vi "example_02_convert.vi"() -> ()   [LabVIEW 2015, in "lv-unit-conversion.lvlib"]
uses:
  lv-unit-conversion.lvlib
  public/_controls/unit.ctl
panel:
  out "error out":errorcluster
  in  "units []":T1[](array[typedef])=[{"symbol"="%", "name"="percent", "dimension"="1", "is_si_unit"=TRUE, "category"="atom-allowed", "base_unit"="Euc", "conversion_reference"="NIST-SI", "is_exact"=TRUE, "a"=0.0, "b"=0.01, "c"=1.0, "d"=0.0, "underlying_def"="1/100 Euc", "description"="Parts per hundred. \n\t\t\t\tThis is one of the few symbols which can be used with multiple unit classes. \n\t\t\t\tIt can be used with each class that represent a ratio of like quantities (e.g., mass per mass).\n\t\t\t"}, {"symbol"="ppk", "name"="part per thousand", "dimension"="1", "is_si_unit"=TRUE, "category"="atom", "base_unit"="Euc", "conversion_reference"="DEFINITION", "is_exact"=TRUE, "a"=0.0, "b"=0.001, "c"=1.0, "d"=0.0, "underlying_def"="", "description"="A ratio of values divided by 1000 where the original values were in the same units."}, {"symbol"="ppm", "name"="part per million", "dimension"="1", "is_si_unit"=TRUE, "category"="atom", "base_unit"="Euc", "conversion_reference"="DEFINITION", "is_exact"=TRUE, "a"=0.0, "b"=1e-06, "c"=1.0, "d"=0.0, "underlying_def"="", "description"="A ratio of values divided by 1E6 where the original values were in the same units."}, {"symbol"="Euc", "name"="euclid", "dimension"="1", "is_si_unit"=TRUE, "category"="atom-allowed", "base_unit"="", "conversion_reference"="", "is_exact"=FALSE, "a"=0.0, "b"=0.0, "c"=0.0, "d"=0.0, "underlying_def"="", "description"="A dimensionless unit of proportion, named after the Greek mathematician, Euclid. \n\t\t\t\tIt represents the SI implied unit of \"1\" which is sometimes called a \"dimensionless derived unit\".\n\t\t\t"}, {"symbol"="byte", "name"="byte", "dimension"="1", "is_si_unit"=TRUE, "category"="atom", "base_unit"="bit", "conversion_reference"="DEFINITION", "is_exact"=TRUE, "a"=0.0, "b"=8.0, "c"=1.0, "d"=0.0, "underlying_def"="8 bit", "description"="8 bit byte."}, {"symbol"="bit", "name"="bit", "dimension"="1", "is_si_unit"=TRUE, "category"="atom-allowed", "base_unit"="", "conversion_reference"="", "is_exact"=FALSE, "a"=0.0, "b"=0.0, "c"=0.0, "d"=0.0, "underlying_def"="Euc", "description"="A bit (a contraction of binary digit) is the basic unit of information in computing and \n\t\t\t\ttelecommunications. \n\t\t\t\tA bit can have only two values: either 1 or 0.\n\t\t\t"}, {"symbol"="%[mass]", "name"="percent [mass basis]", "dimension"="1", "is_si_unit"=TRUE, "category"="atom", "base_unit"="kg/kg", "conversion_reference"="DEFINITION", "is_exact"=TRUE, "a"=0.0, "b"=0.01, "c"=1.0, "d"=0.0, "underlying_def"="", "description"="The percent of mass relative to mass. \n\t\t\t\tThat is, mass divided by mass divided 100 where the original mass values were in the same units.\n\t\t\t"}, {"symbol"="ppm[mass]", "name"="part per million [mass basis]", "dimension"="1", "is_si_unit"=TRUE, "category"="atom", "base_unit"="kg/kg", "conversion_reference"="DEFINITION", "is_exact"=TRUE, "a"=0.0, "b"=1e-06, "c"=1.0, "d"=0.0, "underlying_def"="1E-6 kg/kg", "description"="The parts per million of mass relative to mass. \n\t\t\t\tThat is, mass divided by mass divided by 1E6 where the original mass values were in the same units.\n\t\t\t"}, {"symbol"="%[area]", "name"="percent [area basis]", "dimension"="1", "is_si_unit"=TRUE, "category"="atom", "base_unit"="m2/m2", "conversion_reference"="DERIVED", "is_exact"=TRUE, "a"=0.0, "b"=0.01, "c"=1.0, "d"=0.0, "underlying_def"="", "description"=""}, {"symbol"="%[vol]", "name"="percent [volume basis]", "dimension"="1", "is_si_unit"=TRUE, "category"="atom", "base_unit"="m3/m3", "conversion_reference"="DEFINITION", "is_exact"=TRUE, "a"=0.0, "b"=0.01, "c"=1.0, "d"=0.0, "underlying_def"="1/100 m3/m3", "description"="The percent of volume relative to volume That is, volume divided by volume divided by 100 where the \n\t\t\t\toriginal volume values were in the same units.\n\t\t\t"}, {"symbol"="ppm[vol]", "name"="part per million [volume basis]", "dimension"="1", "is_si_unit"=TRUE, "category"="atom", "base_unit"="m3/m3", "conversion_reference"="DEFINITION", "is_exact"=TRUE, "a"=0.0, "b"=1e-06, "c"=1.0, "d"=0.0, "underlying_def"="1E-6 m3/m3", "description"="The parts per million of volume relative to volume That is, volume divided by volume divided by 1E6 \n\t\t\t\twhere the original volume values were in the same units.\n\t\t\t"}, {"symbol"="%[molar]", "name"="percent [molar basis]", "dimension"="1", "is_si_unit"=TRUE, "category"="atom", "base_unit"="mol/mol", "conversion_reference"="DERIVED", "is_exact"=TRUE, "a"=0.0, "b"=0.01, "c"=1.0, "d"=0.0, "underlying_def"="", "description"=""}, {"symbol"="(bbl/d)/(bbl/d)", "name"="(barrel per day) per (barrel per day)", "dimension"="1", "is_si_unit"=TRUE, "category"="derived", "base_unit"="(m3/s)/(m3/s)", "conversion_reference"="DERIVED", "is_exact"=TRUE, "a"=0.0, "b"=1.0, "c"=1.0, "d"=0.0, "underlying_def"="", "description"=""}, {"symbol"="(m3/d)/(m3/d)", "name"="(cubic metre per day) per (cubic metre per day)", "dimension"="1", "is_si_unit"=TRUE, "category"="derived", "base_unit"="(m3/s)/(m3/s)", "conversion_reference"="DERIVED", "is_exact"=TRUE, "a"=0.0, "b"=1.0, "c"=1.0, "d"=0.0, "underlying_def"="", "description"=""}, {"symbol"="1E6 (ft3/d)/(bbl/d)", "name"="(million cubic foot per day) per (barrel per day)", "dimension"="1", "is_si_unit"=TRUE, "category"="derived", "base_unit"="(m3/s)/(m3/s)", "conversion_reference"="DERIVED", "is_exact"=TRUE, "a"=0.0, "b"=28316.846592, "c"=0.158987294928, "d"=0.0, "underlying_def"="", "description"=""}, {"symbol"="(m3/s)/(m3/s)", "name"="(cubic metre per second) per (cubic metre per second)", "dimension"="1", "is_si_unit"=TRUE, "category"="derived", "base_unit"="", "conversion_reference"="", "is_exact"=FALSE, "a"=0.0, "b"=0.0, "c"=0.0, "d"=0.0, "underlying_def"="Euc", "description"=""}, {"symbol"="kg/kg", "name"="kilogram per kilogram", "dimension"="1", "is_si_unit"=TRUE, "category"="derived", "base_unit"="", "conversion_reference"="", "is_exact"=FALSE, "a"=0.0, "b"=0.0, "c"=0.0, "d"=0.0, "underlying_def"="Euc", "description"=""}, {"symbol"="m/m", "name"="metre per metre", "dimension"="1", "is_si_unit"=TRUE, "category"="derived", "base_unit"="", "conversion_reference"="", "is_exact"=FALSE, "a"=0.0, "b"=0.0, "c"=0.0, "d"=0.0, "underlying_def"="Euc", "description"=""}, {"symbol"="m2/m2", "name"="square metre per square metre", "dimension"="1", "is_si_unit"=TRUE, "category"="derived", "base_unit"="", "conversion_reference"="", "is_exact"=FALSE, "a"=0.0, "b"=0.0, "c"=0.0, "d"=0.0, "underlying_def"="Euc", "description"=""}, {"symbol"="m3/m3", "name"="cubic metre per cubic metre", "dimension"="1", "is_si_unit"=TRUE, "category"="derived", "base_unit"="", "conversion_reference"="", "is_exact"=FALSE, "a"=0.0, "b"=0.0, "c"=0.0, "d"=0.0, "underlying_def"="Euc", "description"=""}, {"symbol"="mol/mol", "name"="mole per mole", "dimension"="1", "is_si_unit"=TRUE, "category"="derived", "base_unit"="", "conversion_reference"="", "is_exact"=FALSE, "a"=0.0, "b"=0.0, "c"=0.0, "d"=0.0, "underlying_def"="Euc", "description"=""}, {"symbol"="N/N", "name"="newton per newton", "dimension"="1", "is_si_unit"=TRUE, "category"="derived", "base_unit"="", "conversion_reference"="", "is_exact"=FALSE, "a"=0.0, "b"=0.0, "c"=0.0, "d"=0.0, "underlying_def"="Euc", "description"=""}, {"symbol"="s/s", "name"="second per second", "dimension"="1", "is_si_unit"=TRUE, "category"="derived", "base_unit"="", "conversion_reference"="", "is_exact"=FALSE, "a"=0.0, "b"=0.0, "c"=0.0, "d"=0.0, "underlying_def"="Euc", "description"=""}, {"symbol"="W/W", "name"="watt per watt", "dimension"="1", "is_si_unit"=TRUE, "category"="derived", "base_unit"="", "conversion_reference"="", "is_exact"=FALSE, "a"=0.0, "b"=0.0, "c"=0.0, "d"=0.0, "underlying_def"="Euc", "description"=""}, {"symbol"="g/kg", "name"="gram per kilogram", "dimension"="1", "is_si_unit"=TRUE, "category"="derived", "base_unit"="kg/kg", "conversion_reference"="DERIVED", "is_exact"=TRUE, "a"=0.0, "b"=0.001, "c"=1.0, "d"=0.0, "underlying_def"="", "description"=""}, {"symbol"="g/t", "name"="gram per tonne", "dimension"="1", "is_si_unit"=TRUE, "category"="derived", "base_unit"="kg/kg", "conversion_reference"="DERIVED", "is_exact"=TRUE, "a"=0.0, "b"=1e-06, "c"=1.0, "d"=0.0, "underlying_def"="", "description"=""}, {"symbol"="kg/sack[94lbm]", "name"="kilogram per 94-pound-sack", "dimension"="1", "is_si_unit"=TRUE, "category"="derived", "base_unit"="kg/kg", "conversion_reference"="DERIVED", "is_exact"=TRUE, "a"=0.0, "b"=1.0, "c"=42.63768278, "d"=0.0, "underlying_def"="", "description"=""}, {"symbol"="kg/t", "name"="kilogram per tonne", "dimension"="1", "is_si_unit"=TRUE, "category"="derived", "base_unit"="kg/kg", "conversion_reference"="DERIVED", "is_exact"=TRUE, "a"=0.0, "b"=0.001, "c"=1.0, "d"=0.0, "underlying_def"="", "description"=""}, {"symbol"="mg/g", "name"="milligram per gram", "dimension"="1", "is_si_unit"=TRUE, "category"="derived", "base_unit"="kg/kg", "conversion_reference"="DERIVED", "is_exact"=TRUE, "a"=0.0, "b"=0.001, "c"=1.0, "d"=0.0, "underlying_def"="", "description"=""}, {"symbol"="mg/kg", "name"="milligram per kilogram", "dimension"="1", "is_si_unit"=TRUE, "category"="derived", "base_unit"="kg/kg", "conversion_reference"="DERIVED", "is_exact"=TRUE, "a"=0.0, "b"=1e-06, "c"=1.0, "d"=0.0, "underlying_def"="", "description"=""}, {"symbol"="ng/g", "name"="nanogram per gram", "dimension"="1", "is_si_unit"=TRUE, "category"="derived", "base_unit"="kg/kg", "conversion_reference"="DERIVED", "is_exact"=TRUE, "a"=0.0, "b"=1e-09, "c"=1.0, "d"=0.0, "underlying_def"="", "description"=""}, {"symbol"="ng/mg", "name"="nanogram per milligram", "dimension"="1", "is_si_unit"=TRUE, "category"="derived", "base_unit"="kg/kg", "conversion_reference"="DERIVED", "is_exact"=TRUE, "a"=0.0, "b"=1e-06, "c"=1.0, "d"=0.0, "underlying_def"="", "description"=""}, {"symbol"="ug/g", "name"="microgram per gram", "dimension"="1", "is_si_unit"=TRUE, "category"="derived", "base_unit"="kg/kg", "conversion_reference"="DERIVED", "is_exact"=TRUE, "a"=0.0, "b"=1e-06, "c"=1.0, "d"=0.0, "underlying_def"="", "description"=""}, {"symbol"="ug/mg", "name"="microgram per milligram", "dimension"="1", "is_si_unit"=TRUE, "category"="derived", "base_unit"="kg/kg", "conversion_reference"="DERIVED", "is_exact"=TRUE, "a"=0.0, "b"=0.001, "c"=1.0, "d"=0.0, "underlying_def"="", "description"=""}, {"symbol"="0.01 ft/ft", "name"="foot per hundred foot", "dimension"="1", "is_si_unit"=TRUE, "category"="derived", "base_unit"="m/m", "conversion_reference"="DERIVED", "is_exact"=TRUE, "a"=0.0, "b"=0.01, "c"=1.0, "d"=0.0, "underlying_def"="", "description"=""}, {"symbol"="1/30 m/m", "name"="metre per thirty metre", "dimension"="1", "is_si_unit"=TRUE, "category"="derived", "base_unit"="m/m", "conversion_reference"="DERIVED", "is_exact"=TRUE, "a"=0.0, "b"=1.0, "c"=30.0, "d"=0.0, "underlying_def"="", "description"=""}, {"symbol"="ft/ft", "name"="foot per foot", "dimension"="1", "is_si_unit"=TRUE, "category"="derived", "base_unit"="m/m", "conversion_reference"="DERIVED", "is_exact"=TRUE, "a"=0.0, "b"=1.0, "c"=1.0, "d"=0.0, "underlying_def"="", "description"=""}, {"symbol"="ft/in", "name"="foot per inch", "dimension"="1", "is_si_unit"=TRUE, "category"="derived", "base_unit"="m/m", "conversion_reference"="DERIVED", "is_exact"=TRUE, "a"=0.0, "b"=12.0, "c"=1.0, "d"=0.0, "underlying_def"="", "description"=""}, {"symbol"="ft/m", "name"="foot per metre", "dimension"="1", "is_si_unit"=TRUE, "category"="derived", "base_unit"="m/m", "conversion_reference"="DERIVED", "is_exact"=TRUE, "a"=0.0, "b"=0.3048, "c"=1.0, "d"=0.0, "underlying_def"="", "description"=""}, {"symbol"="ft/mi", "name"="foot per mile", "dimension"="1", "is_si_unit"=TRUE, "category"="derived", "base_unit"="m/m", "conversion_reference"="DERIVED", "is_exact"=TRUE, "a"=0.0, "b"=1.0, "c"=5280.0, "d"=0.0, "underlying_def"="", "description"=""}, {"symbol"="km/cm", "name"="kilometre per centimetre", "dimension"="1", "is_si_unit"=TRUE, "category"="derived", "base_unit"="m/m", "conversion_reference"="DERIVED", "is_exact"=TRUE, "a"=0.0, "b"=100000.0, "c"=1.0, "d"=0.0, "underlying_def"="", "description"=""}, {"symbol"="m/cm", "name"="metre per centimetre", "dimension"="1", "is_si_unit"=TRUE, "category"="derived", "base_unit"="m/m", "conversion_reference"="DERIVED", "is_exact"=TRUE, "a"=0.0, "b"=100.0, "c"=1.0, "d"=0.0, "underlying_def"="", "description"=""}, {"symbol"="m/km", "name"="metre per kilometre", "dimension"="1", "is_si_unit"=TRUE, "category"="derived", "base_unit"="m/m", "conversion_reference"="DERIVED", "is_exact"=TRUE, "a"=0.0, "b"=0.001, "c"=1.0, "d"=0.0, "underlying_def"="", "description"="Parts per thousand."}, {"symbol"="mi/in", "name"="mile per inch", "dimension"="1", "is_si_unit"=TRUE, "category"="derived", "base_unit"="m/m", "conversion_reference"="DERIVED", "is_exact"=TRUE, "a"=0.0, "b"=63360.0, "c"=1.0, "d"=0.0, "underlying_def"="", "description"=""}, {"symbol"="in2/ft2", "name"="square inch per square foot", "dimension"="1", "is_si_unit"=TRUE, "category"="derived", "base_unit"="m2/m2", "conversion_reference"="DERIVED", "is_exact"=TRUE, "a"=0.0, "b"=1.0, "c"=144.0, "d"=0.0, "underlying_def"="", "description"=""}, {"symbol"="in2/in2", "name"="square inch per square inch", "dimension"="1", "is_si_unit"=TRUE, "category"="derived", "base_unit"="m2/m2", "conversion_reference"="DERIVED", "is_exact"=TRUE, "a"=0.0, "b"=1.0, "c"=1.0, "d"=0.0, "underlying_def"="", "description"=""}, {"symbol"="mm2/mm2", "name"="square millimetre per square millimetre", "dimension"="1", "is_si_unit"=TRUE, "category"="derived", "base_unit"="m2/m2", "conversion_reference"="DERIVED", "is_exact"=TRUE, "a"=0.0, "b"=1.0, "c"=1.0, "d"=0.0, "underlying_def"="", "description"=""}, {"symbol"="0.001 bbl/ft3", "name"="barrel per thousand cubic foot", "dimension"="1", "is_si_unit"=TRUE, "category"="derived", "base_unit"="m3/m3", "conversion_reference"="DERIVED", "is_exact"=TRUE, "a"=0.0, "b"=0.000158987294928, "c"=0.028316846592, "d"=0.0, "underlying_def"="", "description"=""}, {"symbol"="0.001 bbl/m3", "name"="barrel per thousand cubic metre", "dimension"="1", "is_si_unit"=TRUE, "category"="derived", "base_unit"="m3/m3", "conversion_reference"="DERIVED", "is_exact"=TRUE, "a"=0.0, "b"=0.000158987294928, "c"=1.0, "d"=0.0, "underlying_def"="", "description"=""}, {"symbol"="0.001 gal[UK]/bbl", "name"="UK gallon per thousand barrel", "dimension"="1", "is_si_unit"=TRUE, "category"="derived", "base_unit"="m3/m3", "conversion_reference"="DERIVED", "is_exact"=TRUE, "a"=0.0, "b"=4.54609e-06, "c"=0.158987294928, "d"=0.0, "underlying_def"="", "description"=""}, {"symbol"="0.001 gal[UK]/gal[UK]", "name"="UK gallon per thousand UK gallon", "dimension"="1", "is_si_unit"=TRUE, "category"="derived", "base_unit"="m3/m3", "conversion_reference"="DERIVED", "is_exact"=TRUE, "a"=0.0, "b"=0.001, "c"=1.0, "d"=0.0, "underlying_def"="", "description"=""}, {"symbol"="0.001 gal[US]/bbl", "name"="US gallon per thousand barrel", "dimension"="1", "is_si_unit"=TRUE, "category"="derived", "base_unit"="m3/m3", "conversion_reference"="DERIVED", "is_exact"=TRUE, "a"=0.0, "b"=3.785411784e-06, "c"=0.158987294928, "d"=0.0, "underlying_def"="", "description"=""}, {"symbol"="0.001 gal[US]/ft3", "name"="US gallon per thousand cubic foot", "dimension"="1", "is_si_unit"=TRUE, "category"="derived", "base_unit"="m3/m3", "conversion_reference"="DERIVED", "is_exact"=TRUE, "a"=0.0, "b"=3.785411784e-06, "c"=0.028316846592, "d"=0.0, "underlying_def"="", "description"=""}, {"symbol"="0.001 gal[US]/gal[US]", "name"="US gallon per thousand US gallon", "dimension"="1", "is_si_unit"=TRUE, "category"="derived", "base_unit"="m3/m3", "conversion_reference"="DERIVED", "is_exact"=TRUE, "a"=0.0, "b"=0.001, "c"=1.0, "d"=0.0, "underlying_def"="", "description"=""}, {"symbol"="0.001 pt[UK]/bbl", "name"="UK pint per thousand barrel", "dimension"="1", "is_si_unit"=TRUE, "category"="derived", "base_unit"="m3/m3", "conversion_reference"="DERIVED", "is_exact"=TRUE, "a"=0.0, "b"=0.00056826125, "c"=158.987294928, "d"=0.0, "underlying_def"="", "description"=""}, {"symbol"="0.01 bbl/bbl", "name"="barrel per hundred barrel", "dimension"="1", "is_si_unit"=TRUE, "category"="derived", "base_unit"="m3/m3", "conversion_reference"="DERIVED", "is_exact"=TRUE, "a"=0.0, "b"=0.01, "c"=1.0, "d"=0.0, "underlying_def"="", "description"=""}, {"symbol"="0.1 gal[US]/bbl", "name"="US gallon per ten barrel", "dimension"="1", "is_si_unit"=TRUE, "category"="derived", "base_unit"="m3/m3", "conversion_reference"="DERIVED", "is_exact"=TRUE, "a"=0.0, "b"=0.0003785411784, "c"=0.158987294928, "d"=0.0, "underlying_def"="", "description"=""}, {"symbol"="0.1 L/bbl", "name"="litre per ten barrel", "dimension"="1", "is_si_unit"=TRUE, "category"="derived", "base_unit"="m3/m3", "conversion_reference"="DERIVED", "is_exact"=TRUE, "a"=0.0, "b"=0.001, "c"=1.58987294928, "d"=0.0, "underlying_def"="", "description"=""}, {"symbol"="0.1 pt[US]/bbl", "name"="US pint per ten barrel", "dimension"="1", "is_si_unit"=TRUE, "category"="derived", "base_unit"="m3/m3", "conversion_reference"="DERIVED", "is_exact"=TRUE, "a"=0.0, "b"=0.000473176473, "c"=1.58987294928, "d"=0.0, "underlying_def"="", "description"=""}, {"symbol"="1000 ft3/bbl", "name"="thousand cubic foot per barrel", "dimension"="1", "is_si_unit"=TRUE, "category"="derived", "base_unit"="m3/m3", "conversion_reference"="DERIVED", "is_exact"=TRUE, "a"=0.0, "b"=28.316846592, "c"=0.158987294928, "d"=0.0, "underlying_def"="", "description"=""}, {"symbol"="1000 m3/m3", "name"="thousand cubic metre per cubic metre", "dimension"="1", "is_si_unit"=TRUE, "category"="derived", "base_unit"="m3/m3", "conversion_reference"="DERIVED", "is_exact"=TRUE, "a"=0.0, "b"=1000.0, "c"=1.0, "d"=0.0, "underlying_def"="", "description"=""}, {"symbol"="1E-6 acre.ft/bbl", "name"="acre foot per million barrel", "dimension"="1", "is_si_unit"=TRUE, "category"="derived", "base_unit"="m3/m3", "conversion_reference"="DERIVED", "is_exact"=TRUE, "a"=0.0, "b"=19119.00672, "c"=2464298.1427778574, "d"=0.0, "underlying_def"="", "description"=""}, {"symbol"="1E6 bbl/(acre.ft)", "name"="million barrel per acre foot", "dimension"="1", "is_si_unit"=TRUE, "category"="derived", "base_unit"="m3/m3", "conversion_reference"="DERIVED", "is_exact"=TRUE, "a"=0.0, "b"=2464298142777.8574, "c"=19119006720.0, "d"=0.0, "underlying_def"="", "description"=""}, {"symbol"="1E-6 bbl/ft3", "name"="barrel per million cubic foot", "dimension"="1", "is_si_unit"=TRUE, "category"="derived", "base_unit"="m3/m3", "conversion_reference"="DERIVED", "is_exact"=TRUE, "a"=0.0, "b"=0.158987294928, "c"=28316.846592, "d"=0.0, "underlying_def"="", "description"=""}, {"symbol"="1E-6 bbl/m3", "name"="barrel per million cubic metre", "dimension"="1", "is_si_unit"=TRUE, "category"="derived", "base_unit"="m3/m3", "conversion_reference"="DERIVED", "is_exact"=TRUE, "a"=0.0, "b"=1.58987294928e-07, "c"=1.0, "d"=0.0, "underlying_def"="", "description"="barrel per million cubic metre"}, {"symbol"="1E6 ft3/(acre.ft)", "name"="million cubic foot per acre foot", "dimension"="1", "is_si_unit"=TRUE, "category"="derived", "base_unit"="m3/m3", "conversion_reference"="DERIVED", "is_exact"=TRUE, "a"=0.0, "b"=1439994240005.76, "c"=62726400000.0, "d"=0.0, "underlying_def"="", "description"=""}, {"symbol"="1E6 ft3/bbl", "name"="million cubic foot per barrel", "dimension"="1", "is_si_unit"=TRUE, "category"="derived", "base_unit"="m3/m3", "conversion_reference"="DERIVED", "is_exact"=TRUE, "a"=0.0, "b"=28316.846592, "c"=0.158987294928, "d"=0.0, "underlying_def"="", "description"=""}, {"symbol"="bbl/(acre.ft)", "name"="barrel per acre foot", "dimension"="1", "is_si_unit"=TRUE, "category"="derived", "base_unit"="m3/m3", "conversion_reference"="DERIVED", "is_exact"=TRUE, "a"=0.0, "b"=2464298.1427778574, "c"=19119006720.0, "d"=0.0, "underlying_def"="", "description"=""}, {"symbol"="bbl/bbl", "name"="barrel per barrel", "dimension"="1", "is_si_unit"=TRUE, "category"="derived", "base_unit"="m3/m3", "conversion_reference"="DERIVED", "is_exact"=TRUE, "a"=0.0, "b"=1.0, "c"=1.0, "d"=0.0, "underlying_def"="", "description"=""}, {"symbol"="bbl/ft3", "name"="barrel per cubic foot", "dimension"="1", "is_si_unit"=TRUE, "category"="derived", "base_unit"="m3/m3", "conversion_reference"="DERIVED", "is_exact"=TRUE, "a"=0.0, "b"=0.158987294928, "c"=0.028316846592, "d"=0.0, "underlying_def"="", "description"=""}, {"symbol"="bbl/m3", "name"="barrel per cubic metre", "dimension"="1", "is_si_unit"=TRUE, "category"="derived", "base_unit"="m3/m3", "conversion_reference"="DERIVED", "is_exact"=TRUE, "a"=0.0, "b"=0.158987294928, "c"=1.0, "d"=0.0, "underlying_def"="", "description"=""}, {"symbol"="cm3/cm3", "name"="cubic centimetre per cubic centimetre", "dimension"="1", "is_si_unit"=TRUE, "category"="derived", "base_unit"="m3/m3", "conversion_reference"="DERIVED", "is_exact"=TRUE, "a"=0.0, "b"=1.0, "c"=1.0, "d"=0.0, "underlying_def"="", "description"=""}, {"symbol"="cm3/L", "name"="cubic centimetre per litre", "dimension"="1", "is_si_unit"=TRUE, "category"="derived", "base_unit"="m3/m3", "conversion_reference"="DERIVED", "is_exact"=TRUE, "a"=0.0, "b"=0.001, "c"=1.0, "d"=0.0, "underlying_def"="", "description"=""}, {"symbol"="cm3/m3", "name"="cubic centimetre per cubic metre", "dimension"="1", "is_si_unit"=TRUE, "category"="derived", "base_unit"="m3/m3", "conversion_reference"="DERIVED", "is_exact"=TRUE, "a"=0.0, "b"=1e-06, "c"=1.0, "d"=0.0, "underlying_def"="", "description"="Part per million [mass per mass]"}, {"symbol"="dm3/m3", "name"="cubic decimetre per cubic metre", "dimension"="1", "is_si_unit"=TRUE, "category"="derived", "base_unit"="m3/m3", "conversion_reference"="DERIVED", "is_exact"=TRUE, "a"=0.0, "b"=0.001, "c"=1.0, "d"=0.0, "underlying_def"="", "description"=""}, {"symbol"="ft3/bbl", "name"="cubic foot per barrel", "dimension"="1", "is_si_unit"=TRUE, "category"="derived", "base_unit"="m3/m3", "conversion_reference"="DERIVED", "is_exact"=TRUE, "a"=0.0, "b"=0.028316846592, "c"=0.158987294928, "d"=0.0, "underlying_def"="", "description"=""}, {"symbol"="ft3/ft3", "name"="cubic foot per cubic foot", "dimension"="1", "is_si_unit"=TRUE, "category"="derived", "base_unit"="m3/m3", "conversion_reference"="DERIVED", "is_exact"=TRUE, "a"=0.0, "b"=1.0, "c"=1.0, "d"=0.0, "underlying_def"="", "description"=""}, {"symbol"="gal[UK]/ft3", "name"="UK gallon per cubic foot", "dimension"="1", "is_si_unit"=TRUE, "category"="derived", "base_unit"="m3/m3", "conversion_reference"="DERIVED", "is_exact"=TRUE, "a"=0.0, "b"=0.00454609, "c"=0.028316846592, "d"=0.0, "underlying_def"="", "description"=""}, {"symbol"="gal[US]/bbl", "name"="US gallon per barrel", "dimension"="1", "is_si_unit"=TRUE, "category"="derived", "base_unit"="m3/m3", "conversion_reference"="DERIVED", "is_exact"=TRUE, "a"=0.0, "b"=0.003785411784, "c"=0.158987294928, "d"=0.0, "underlying_def"="", "description"=""}, {"symbol"="gal[US]/ft3", "name"="US gallon per cubic foot", "dimension"="1", "is_si_unit"=TRUE, "category"="derived", "base_unit"="m3/m3", "conversion_reference"="DERIVED", "is_exact"=TRUE, "a"=0.0, "b"=0.003785411784, "c"=0.028316846592, "d"=0.0, "underlying_def"="", "description"=""}, {"symbol"="L/m3", "name"="litre per cubic metre", "dimension"="1", "is_si_unit"=TRUE, "category"="derived", "base_unit"="m3/m3", "conversion_reference"="DERIVED", "is_exact"=TRUE, "a"=0.0, "b"=0.001, "c"=1.0, "d"=0.0, "underlying_def"="", "description"=""}, {"symbol"="m3/(ha.m)", "name"="cubic metre per hectare metre", "dimension"="1", "is_si_unit"=TRUE, "category"="derived", "base_unit"="m3/m3", "conversion_reference"="DERIVED", "is_exact"=TRUE, "a"=0.0, "b"=0.0001, "c"=1.0, "d"=0.0, "underlying_def"="", "description"=""}, {"symbol"="m3/bbl", "name"="cubic metre per barrel", "dimension"="1", "is_si_unit"=TRUE, "category"="derived", "base_unit"="m3/m3", "conversion_reference"="DERIVED", "is_exact"=TRUE, "a"=0.0, "b"=1.0, "c"=0.158987294928, "d"=0.0, "underlying_def"="", "description"=""}, {"symbol"="mL/gal[UK]", "name"="millilitre per UK gallon", "dimension"="1", "is_si_unit"=TRUE, "category"="derived", "base_unit"="m3/m3", "conversion_reference"="DERIVED", "is_exact"=TRUE, "a"=0.0, "b"=1e-06, "c"=0.00454609, "d"=0.0, "underlying_def"="", "description"=""}, {"symbol"="mL/gal[US]", "name"="millilitre per US gallon", "dimension"="1", "is_si_unit"=TRUE, "category"="derived", "base_unit"="m3/m3", "conversion_reference"="DERIVED", "is_exact"=TRUE, "a"=0.0, "b"=1e-06, "c"=0.003785411784, "d"=0.0, "underlying_def"="", "description"=""}, {"symbol"="mL/mL", "name"="millilitre per millilitre", "dimension"="1", "is_si_unit"=TRUE, "category"="derived", "base_unit"="m3/m3", "conversion_reference"="DERIVED", "is_exact"=TRUE, "a"=0.0, "b"=1.0, "c"=1.0, "d"=0.0, "underlying_def"="", "description"=""}, {"symbol"="kgf/kgf", "name"="thousand gram-force per kilogram-force", "dimension"="1", "is_si_unit"=TRUE, "category"="derived", "base_unit"="N/N", "conversion_reference"="DERIVED", "is_exact"=TRUE, "a"=0.0, "b"=1.0, "c"=1.0, "d"=0.0, "underlying_def"="", "description"=""}, {"symbol"="lbf/lbf", "name"="pound-force per pound-force", "dimension"="1", "is_si_unit"=TRUE, "category"="derived", "base_unit"="N/N", "conversion_reference"="DERIVED", "is_exact"=TRUE, "a"=0.0, "b"=1.0, "c"=1.0, "d"=0.0, "underlying_def"="", "description"=""}, {"symbol"="ms/s", "name"="millisecond per second", "dimension"="1", "is_si_unit"=TRUE, "category"="derived", "base_unit"="s/s", "conversion_reference"="DERIVED", "is_exact"=TRUE, "a"=0.0, "b"=0.001, "c"=1.0, "d"=0.0, "underlying_def"="", "description"=""}, {"symbol"="Btu[IT]/(hp.h)", "name"="BTU per horsepower hour", "dimension"="1", "is_si_unit"=TRUE, "category"="derived", "base_unit"="W/W", "conversion_reference"="DERIVED", "is_exact"=TRUE, "a"=0.0, "b"=1055.05585262, "c"=2684519.537696173, "d"=0.0, "underlying_def"="", "description"=""}, {"symbol"="W/kW", "name"="watt per kilowatt", "dimension"="1", "is_si_unit"=TRUE, "category"="derived", "base_unit"="W/W", "conversion_reference"="DERIVED", "is_exact"=TRUE, "a"=0.0, "b"=0.001, "c"=1.0, "d"=0.0, "underlying_def"="", "description"=""}, {"symbol"="cEuc", "name"="centieuclid", "dimension"="1", "is_si_unit"=TRUE, "category"="prefixed", "base_unit"="Euc", "conversion_reference"="DERIVED", "is_exact"=TRUE, "a"=0.0, "b"=0.01, "c"=1.0, "d"=0.0, "underlying_def"="", "description"="Parts per hundred."}, {"symbol"="dEuc", "name"="decieuclid", "dimension"="1", "is_si_unit"=TRUE, "category"="prefixed", "base_unit"="Euc", "conversion_reference"="DERIVED", "is_exact"=TRUE, "a"=0.0, "b"=0.1, "c"=1.0, "d"=0.0, "underlying_def"="", "description"="Parts per ten."}, {"symbol"="EEuc", "name"="exaeuclid", "dimension"="1", "is_si_unit"=TRUE, "category"="prefixed", "base_unit"="Euc", "conversion_reference"="DERIVED", "is_exact"=TRUE, "a"=0.0, "b"=1e+18, "c"=1.0, "d"=0.0, "underlying_def"="", "description"="Million million million per part."}, {"symbol"="fEuc", "name"="femtoeuclid", "dimension"="1", "is_si_unit"=TRUE, "category"="prefixed", "base_unit"="Euc", "conversion_reference"="DERIVED", "is_exact"=TRUE, "a"=0.0, "b"=1e-15, "c"=1.0, "d"=0.0, "underlying_def"="", "description"="Parts per thousand million million."}, {"symbol"="GEuc", "name"="gigaeuclid", "dimension"="1", "is_si_unit"=TRUE, "category"="prefixed", "base_unit"="Euc", "conversion_reference"="DERIVED", "is_exact"=TRUE, "a"=0.0, "b"=1000000000.0, "c"=1.0, "d"=0.0, "underlying_def"="", "description"="Thousand million per part."}, {"symbol"="kEuc", "name"="kiloeuclid", "dimension"="1", "is_si_unit"=TRUE, "category"="prefixed", "base_unit"="Euc", "conversion_reference"="DERIVED", "is_exact"=TRUE, "a"=0.0, "b"=1000.0, "c"=1.0, "d"=0.0, "underlying_def"="", "description"="Thousand per part."}, {"symbol"="mEuc", "name"="millieuclid", "dimension"="1", "is_si_unit"=TRUE, "category"="prefixed", "base_unit"="Euc", "conversion_reference"="DERIVED", "is_exact"=TRUE, "a"=0.0, "b"=0.001, "c"=1.0, "d"=0.0, "underlying_def"="", "description"="Parts per thousand."}, {"symbol"="MEuc", "name"="megaeuclid", "dimension"="1", "is_si_unit"=TRUE, "category"="prefixed", "base_unit"="Euc", "conversion_reference"="DERIVED", "is_exact"=TRUE, "a"=0.0, "b"=1000000.0, "c"=1.0, "d"=0.0, "underlying_def"="", "description"="Million per part."}, {"symbol"="nEuc", "name"="nanoeuclid", "dimension"="1", "is_si_unit"=TRUE, "category"="prefixed", "base_unit"="Euc", "conversion_reference"="DERIVED", "is_exact"=TRUE, "a"=0.0, "b"=1e-09, "c"=1.0, "d"=0.0, "underlying_def"="", "description"="Parts per thousand million."}, {"symbol"="pEuc", "name"="picoeuclid", "dimension"="1", "is_si_unit"=TRUE, "category"="prefixed", "base_unit"="Euc", "conversion_reference"="DERIVED", "is_exact"=TRUE, "a"=0.0, "b"=1e-12, "c"=1.0, "d"=0.0, "underlying_def"="", "description"="Parts per million million."}, {"symbol"="TEuc", "name"="teraeuclid", "dimension"="1", "is_si_unit"=TRUE, "category"="prefixed", "base_unit"="Euc", "conversion_reference"="DERIVED", "is_exact"=TRUE, "a"=0.0, "b"=1000000000000.0, "c"=1.0, "d"=0.0, "underlying_def"="", "description"="Million million per part."}, {"symbol"="uEuc", "name"="microeuclid", "dimension"="1", "is_si_unit"=TRUE, "category"="prefixed", "base_unit"="Euc", "conversion_reference"="EPSG", "is_exact"=TRUE, "a"=0.0, "b"=1e-06, "c"=1.0, "d"=0.0, "underlying_def"="", "description"="Parts per million."}, {"symbol"="Kibyte", "name"="kibibyte", "dimension"="1", "is_si_unit"=TRUE, "category"="prefixed", "base_unit"="bit", "conversion_reference"="DERIVED", "is_exact"=TRUE, "a"=0.0, "b"=8192.0, "c"=1.0, "d"=0.0, "underlying_def"="", "description"="1024 bytes."}, {"symbol"="Mibyte", "name"="mebibyte", "dimension"="1", "is_si_unit"=TRUE, "category"="prefixed", "base_unit"="bit", "conversion_reference"="DERIVED", "is_exact"=TRUE, "a"=0.0, "b"=8388608.0, "c"=1.0, "d"=0.0, "underlying_def"="", "description"="1048576 bytes. \n\t\t\t\tCommonly called a megabyte but mega refers to powers of ten rather than powers of two.\n\t\t\t"}, {"symbol"="1/deltaC", "name"="per delta Celsius", "dimension"="1/D", "is_si_unit"=TRUE, "category"="derived", "base_unit"="1/deltaK", "conversion_reference"="DERIVED", "is_exact"=TRUE, "a"=0.0, "b"=1.0, "c"=1.0, "d"=0.0, "underlying_def"="", "description"=""}, {"symbol"="1/deltaF", "name"="per delta Fahrenheit", "dimension"="1/D", "is_si_unit"=TRUE, "category"="derived", "base_unit"="1/deltaK", "conversion_reference"="DERIVED", "is_exact"=TRUE, "a"=0.0, "b"=9.0, "c"=5.0, "d"=0.0, "underlying_def"="", "description"=""}, {"symbol"="1/deltaR", "name"="per delta Rankine", "dimension"="1/D", "is_si_unit"=TRUE, "category"="derived", "base_unit"="1/deltaK", "conversion_reference"="DERIVED", "is_exact"=TRUE, "a"=0.0, "b"=9.0, "c"=5.0, "d"=0.0, "underlying_def"="", "description"=""}, {"symbol"="1/deltaK", "name"="per delta kelvin", "dimension"="1/D", "is_si_unit"=TRUE, "category"="derived", "base_unit"="", "conversion_reference"="", "is_exact"=FALSE, "a"=0.0, "b"=0.0, "c"=0.0, "d"=0.0, "underlying_def"="", "description"=""}, {"symbol"="m/(m.deltaK)", "name"="metre per metre delta kelvin", "dimension"="1/D", "is_si_unit"=TRUE, "category"="derived", "base_unit"="", "conversion_reference"="", "is_exact"=FALSE, "a"=0.0, "b"=0.0, "c"=0.0, "d"=0.0, "underlying_def"="1/deltaK", "description"=""}, {"symbol"="m3/(m3.deltaK)", "name"="cubic metre per cubic metre delta kelvin", "dimension"="1/D", "is_si_unit"=TRUE, "category"="derived", "base_unit"="", "conversion_reference"="", "is_exact"=FALSE, "a"=0.0, "b"=0.0, "c"=0.0, "d"=0.0, "underlying_def"="1/deltaK", "description"=""}, {"symbol"="in/(in.deltaF)", "name"="inch per inch delta Fahrenheit", "dimension"="1/D", "is_si_unit"=TRUE, "category"="derived", "base_unit"="m/(m.deltaK)", "conversion_reference"="DERIVED", "is_exact"=TRUE, "a"=0.0, "b"=9.0, "c"=5.0, "d"=0.0, "underlying_def"="", "description"=""}, {"symbol"="mm/(mm.deltaK)", "name"="millimetre per millimetre delta kelvin", "dimension"="1/D", "is_si_unit"=TRUE, "category"="derived", "base_unit"="m/(m.deltaK)", "conversion_reference"="DERIVED", "is_exact"=TRUE, "a"=0.0, "b"=1.0, "c"=1.0, "d"=0.0, "underlying_def"="", "description"=""}, {"symbol"="1E-6 m3/(m3.deltaC)", "name"="(cubic metre per million cubic metre) per delta Celsius", "dimension"="1/D", "is_si_unit"=TRUE, "category"="derived", "base_unit"="m3/(m3.deltaK)", "conversion_reference"="DERIVED", "is_exact"=TRUE, "a"=0.0, "b"=1e-06, "c"=1.0, "d"=0.0, "underlying_def"="", "description"=""}, {"symbol"="1E-6 m3/(m3.deltaF)", "name"="(cubic metre per million cubic metre) per delta Fahrenheit", "dimension"="1/D", "is_si_unit"=TRUE, "category"="derived", "base_unit"="m3/(m3.deltaK)", "conversion_reference"="DERIVED", "is_exact"=TRUE, "a"=0.0, "b"=9e-06, "c"=5.0, "d"=0.0, "underlying_def"="", "description"=""}, {"symbol"="ppm[vol]/deltaC", "name"="(part per million [volume basis]) per delta Celsius", "dimension"="1/D", "is_si_unit"=TRUE, "category"="derived", "base_unit"="m3/(m3.deltaK)", "conversion_reference"="DERIVED", "is_exact"=TRUE, "a"=0.0, "b"=1e-06, "c"=1.0, "d"=0.0, "underlying_def"="1E-6 m3/(m3.deltaC)", "description"=""}, {"symbol"="ppm[vol]/deltaF", "name"="(part per million [volume basis)] per delta Fahrenheit", "dimension"="1/D", "is_si_unit"=TRUE, "category"="derived", "base_unit"="m3/(m3.deltaK)", "conversion_reference"="DERIVED", "is_exact"=TRUE, "a"=0.0, "b"=9e-06, "c"=5.0, "d"=0.0, "underlying_def"="1E-6 m3/(m3.deltaF)", "description"=""}, {"symbol"="cu", "name"="capture unit", "dimension"="1/L", "is_si_unit"=TRUE, "category"="atom", "base_unit"="m2/m3", "conversion_reference"="SPE-1984", "is_exact"=TRUE, "a"=0.0, "b"=0.1, "c"=1.0, "d"=0.0, "underlying_def"="1E-3 cm2/cm3", "description"="The macroscopic capture cross section is the sum of all the various weighted elemental capture cross \n\t\t\t\tsections. \n\t\t\t\tThe are \"1E-3 cm2/cm3\" often referred to as capture unit (c.u.) or sigma unit (s.u.). \n\t\t\t\t(Adapted from Ransom, Robert C,\" Practical Formation Evaluation\", New York: J Wiley, 1995.)\n\t\t\t"}, {"symbol"="1/angstrom", "name"="per angstrom", "dimension"="1/L", "is_si_unit"=TRUE, "category"="derived", "base_unit"="1/m", "conversion_reference"="DERIVED", "is_exact"=TRUE, "a"=0.0, "b"=10000000000.0, "c"=1.0, "d"=0.0, "underlying_def"="", "description"=""}, {"symbol"="1/cm", "name"="per centimetre", "dimension"="1/L", "is_si_unit"=TRUE, "category"="derived", "base_unit"="1/m", "conversion_reference"="DERIVED", "is_exact"=TRUE, "a"=0.0, "b"=100.0, "c"=1.0, "d"=0.0, "underlying_def"="", "description"=""}, {"symbol"="1/ft", "name"="per foot", "dimension"="1/L", "is_si_unit"=TRUE, "category"="derived", "base_unit"="1/m", "conversion_reference"="DERIVED", "is_exact"=TRUE, "a"=0.0, "b"=1.0, "c"=0.3048, "d"=0.0, "underlying_def"="", "description"=""}, {"symbol"="1/in", "name"="per inch", "dimension"="1/L", "is_si_unit"=TRUE, "category"="derived", "base_unit"="1/m", "conversion_reference"="DERIVED", "is_exact"=TRUE, "a"=0.0, "b"=1.0, "c"=0.0254, "d"=0.0, "underlying_def"="", "description"=""}, {"symbol"="1/mi", "name"="per mile", "dimension"="1/L", "is_si_unit"=TRUE, "category"="derived", "base_unit"="1/m", "conversion_reference"="DERIVED", "is_exact"=TRUE, "a"=0.0, "b"=1.0, "c"=1609.344, "d"=0.0, "underlying_def"="", "description"=""}, {"symbol"="1/mm", "name"="per millimetre", "dimension"="1/L", "is_si_unit"=TRUE, "category"="derived", "base_unit"="1/m", "conversion_reference"="DERIVED", "is_exact"=TRUE, "a"=0.0, "b"=1000.0, "c"=1.0, "d"=0.0, "underlying_def"="", "description"=""}, {"symbol"="1/nm", "name"="per nanometre", "dimension"="1/L", "is_si_unit"=TRUE, "category"="derived", "base_unit"="1/m", "conversion_reference"="DERIVED", "is_exact"=TRUE, "a"=0.0, "b"=1000000000.0, "c"=1.0, "d"=0.0, "underlying_def"="", "description"=""}, {"symbol"="1/yd", "name"="per yard", "dimension"="1/L", "is_si_unit"=TRUE, "category"="derived", "base_unit"="1/m", "conversion_reference"="DERIVED", "is_exact"=TRUE, "a"=0.0, "b"=1.0, "c"=0.9144, "d"=0.0, "underlying_def"="", "description"=""}, {"symbol"="1E-9 1/ft", "name"="per thousand million foot", "dimension"="1/L", "is_si_unit"=TRUE, "category"="derived", "base_unit"="1/m", "conversion_reference"="DERIVED", "is_exact"=TRUE, "a"=0.0, "b"=1e-09, "c"=0.3048, "d"=0.0, "underlying_def"="", "description"=""}, {"symbol"="b/cm3", "name"="barn per cubic centimetre", "dimension"="1/L", "is_si_unit"=TRUE, "category"="derived", "base_unit"="1/m", "conversion_reference"="DERIVED", "is_exact"=TRUE, "a"=0.0, "b"=1e-22, "c"=1.0, "d"=0.0, "underlying_def"="", "description"=""}, {"symbol"="ft2/in3", "name"="square foot per cubic inch", "dimension"="1/L", "is_si_unit"=TRUE, "category"="derived", "base_unit"="1/m", "conversion_reference"="DERIVED", "is_exact"=TRUE, "a"=0.0, "b"=0.09290304, "c"=1.6387064e-05, "d"=0.0, "underlying_def"="", "description"=""}, {"symbol"="m2/cm3", "name"="square metre per cubic centimetre", "dimension"="1/L", "is_si_unit"=TRUE, "category"="derived", "base_unit"="1/m", "conversion_reference"="DERIVED", "is_exact"=TRUE, "a"=0.0, "b"=1000000.0, "c"=1.0, "d"=0.0, "underlying_def"="", "description"=""}, {"symbol"="1/m", "name"="per metre", "dimension"="1/L", "is_si_unit"=TRUE, "category"="derived", "base_unit"="", "conversion_reference"="", "is_exact"=FALSE, "a"=0.0, "b"=0.0, "c"=0.0, "d"=0.0, "underlying_def"="", "description"=""}, {"symbol"="m2/m3", "name"="square metre per cubic metre", "dimension"="1/L", "is_si_unit"=TRUE, "category"="derived", "base_unit"="", "conversion_reference"="", "is_exact"=FALSE, "a"=0.0, "b"=0.0, "c"=0.0, "d"=0.0, "underlying_def"="1/m", "description"=""}, {"symbol"="1/ft2", "name"="per square foot", "dimension"="1/L2", "is_si_unit"=TRUE, "category"="derived", "base_unit"="1/m2", "conversion_reference"="DERIVED", "is_exact"=TRUE, "a"=0.0, "b"=1.0, "c"=0.09290304, "d"=0.0, "underlying_def"="", "description"=""}, {"symbol"="1/km2", "name"="per square kilometre", "dimension"="1/L2", "is_si_unit"=TRUE, "category"="derived", "base_unit"="1/m2", "conversion_reference"="DERIVED", "is_exact"=TRUE, "a"=0.0, "b"=1e-06, "c"=1.0, "d"=0.0, "underlying_def"="", "description"=""}, {"symbol"="1/mi2", "name"="per square mile", "dimension"="1/L2", "is_si_unit"=TRUE, "category"="derived", "base_unit"="1/m2", "conversion_reference"="DERIVED", "is_exact"=TRUE, "a"=0.0, "b"=1.0, "c"=2589988.110336, "d"=0.0, "underlying_def"="", "description"=""}, {"symbol"="1/m2", "name"="per square metre", "dimension"="1/L2", "is_si_unit"=TRUE, "category"="derived", "base_unit"="", "conversion_reference"="", "is_exact"=FALSE, "a"=0.0, "b"=0.0, "c"=0.0, "d"=0.0, "underlying_def"="", "description"=""}, {"symbol"="m/m3", "name"="metre per cubic metre", "dimension"="1/L2", "is_si_unit"=TRUE, "category"="derived", "base_unit"="", "conversion_reference"="", "is_exact"=FALSE, "a"=0.0, "b"=0.0, "c"=0.0, "d"=0.0, "underlying_def"="1/m2", "description"=""}, {"symbol"="ft/bbl", "name"="foot per barrel", "dimension"="1/L2", "is_si_unit"=TRUE, "category"="derived", "base_unit"="m/m3", "conversion_reference"="DERIVED", "is_exact"=TRUE, "a"=0.0, "b"=0.3048, "c"=0.158987294928, "d"=0.0, "underlying_def"="", "description"=""}, {"symbol"="ft/ft3", "name"="foot per cubic foot", "dimension"="1/L2", "is_si_unit"=TRUE, "category"="derived", "base_unit"="m/m3", "conversion_reference"="DERIVED", "is_exact"=TRUE, "a"=0.0, "b"=1.0, "c"=0.09290304, "d"=0.0, "underlying_def"="", "description"=""}, {"symbol"="ft/gal[US]", "name"="foot per US gallon", "dimension"="1/L2", "is_si_unit"=TRUE, "category"="derived", "base_unit"="m/m3", "conversion_reference"="DERIVED", "is_exact"=TRUE, "a"=0.0, "b"=0.3048, "c"=0.003785411784, "d"=0.0, "underlying_def"="", "description"=""}, {"symbol"="km/dm3", "name"="kilometre per cubic decimetre", "dimension"="1/L2", "is_si_unit"=TRUE, "category"="derived", "base_unit"="m/m3", "conversion_reference"="DERIVED", "is_exact"=TRUE, "a"=0.0, "b"=1000000.0, "c"=1.0, "d"=0.0, "underlying_def"="", "description"=""}, {"symbol"="km/L", "name"="kilometre per litre", "dimension"="1/L2", 
